vi "deserialize (Messages).vi"(11 "data in":string[][](array[string])) -> (3 "messages":map{string, T1}(c390))   [LabVIEW 2020]
uses:
  _controls/1553_messages.ctl
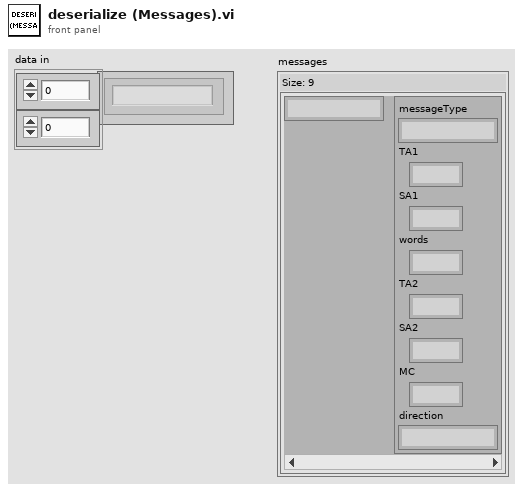
[diagram p1: front panel]
types:
  T1 = typedef "1553_messages.ctl" = cluster{"messageType":string, "TA1":i32, "SA1":i32, "words":i32, "TA2":i32, "SA2":i32, "MC":i32, "direction":string}
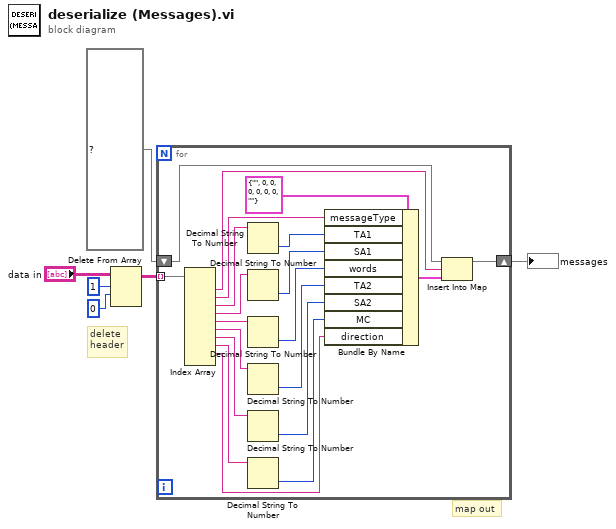
[diagram p0: block diagram]
diagram:
  # "delete\nheader"
  # "map out"
  n1 = Delete From Array(array="data in", length=1, index (row)=0) -> (array with subset deleted=w1:string[][])  [unwired: 1 in, 1 out]
  n2 = for {
    tunnel: w1 -> [w26] mode=indexing
    shift-right: [w21] -> w5
    shift-left: map{string, T1} {} ("map") -> [w24]
    n3 = Index Array(array=w26) -> (element #1=w22:string, element #2=w20:string, element #3=w19:string, element #4=w17:string, element #5=w16:string, element #6=w13:string, element #7=w12:string, element #8=w11:string, element #9=w10:string)  [unwired: 10 in, 1 out]
    n4 = Decimal String To Number(string=w19) -> (number=w18:i32)  [unwired: 2 in, 1 out]
    n5 = Decimal String To Number(string=w17) -> (number=w15:i32)  [unwired: 2 in, 1 out]
    n6 = Decimal String To Number(string=w16) -> (number=w14:i32)  [unwired: 2 in, 1 out]
    n7 = Decimal String To Number(string=w13) -> (number=w9:i32)  [unwired: 2 in, 1 out]
    n8 = Decimal String To Number(string=w12) -> (number=w8:i32)  [unwired: 2 in, 1 out]
    n9 = Decimal String To Number(string=w11) -> (number=w7:i32)  [unwired: 2 in, 1 out]
    n10 = Bundle By Name(cluster=T1 {"messageType"="", "TA1"=0, "SA1"=0, "words"=0, "TA2"=0, "SA2"=0, "MC"=0, "direction"=""}, "messageType"=w20, "TA1"=w18, "SA1"=w15, "words"=w14, "TA2"=w9, "SA2"=w8, "MC"=w7, "direction"=w10) -> (w23:T1)
    n11 = Insert Into Map(map in=w24, key=w22, value=w23) -> (map out=w21:map{string, T1})  [unwired: 2 out]
  }
  "messages" <- w5
